vi "Autonomous Independent.vi"   [LabVIEW 2015]
doc: "This VI is called when autonomous begins, and will automatically be terminated when autonomous ends. You can carry out timed or sensor driven robot movement independently without needing to return to the caller."
uses:
  <vilib>/Rock Robotics/WPI/CAN/TalonSRX/WPI_CANTalonSRX_BrakeOverride.ctl
  <vilib>/Rock Robotics/WPI/Solenoid/WPI_SolenoidValue.ctl
  <vilib>/Analysis/baseanly.llb/Mean (DBL).vi
  <vilib>/Rock Robotics/WPI/Utilities/WPI_GetSetVariantRefNum.vi
  <vilib>/Rock Robotics/Network Tables/NT Write Numeric Array.vi
  <vilib>/Rock Robotics/Network Tables/NT Read Numeric Array.vi
  <vilib>/Rock Robotics/Network Tables/NT Read String Array.vi
  <vilib>/Rock Robotics/Network Tables/NT Write String.vi
  <vilib>/addons/control/pid/pid.llb/PID (DBL).vi
  <vilib>/Rock Robotics/WPI/Solenoid/WPI_SolenoidSetEnum.vi
  <vilib>/addons/control/pid/NI_PID_pid.lvlib
  ADI MXP IMU/ADI MXP IMU/FRC ADI MXP IMU.lvlib
  <vilib>/Analysis/NI_AALBase.lvlib
panel:
  # "Be sure to right-click and choose Data Operations>>Make Current Value default if you want to save the array values with the VI"
types:
  T1 = typedef "WPI_JoystickDevRef.ctl" = cluster{"Device":T2}
  T2 = typedef "WPI_JoystickDeviceEnum.ctl" = enum16{"USB 0", "USB 1", "USB 2", "USB 3", "USB 4", "USB 5"}
  T3 = typedef "WPI_EncoderDevRef.ctl" = cluster{"DevStatus":errorcluster, "EncoderIndex":T4, "CounterIndex":T5, "DistancePerCount":dbl, "Decoding Type":T6}
  T4 = typedef "FPGA_EncoderIdx.ctl" = enum8{"Enc 0", "Enc 1", "Enc 2", "Enc 3", "Enc 4", "Enc 5", "Enc 6", "Enc 7", "Invalid"}
  T5 = typedef "FPGA_CounterCtrSystemIndex.ctl" = enum8{"Ctr 0", "Ctr 1", "Ctr 2", "Ctr 3", "Ctr 4", "Ctr 5", "Ctr 6", "Ctr 7", "Invalid"}
  T6 = typedef "WPI_EncoderType.ctl" = enum16{"1x", "2x", "4x"}
  T7 = cluster{"proportional gain (Kc)":dbl, "integral time (Ti, min)":dbl, "derivative time (Td, min)":dbl}
  T8 = typedef "WPI_SolenoidValue.ctl" = enum16{"Off", "On", "Forward", "Reverse"}
  T9 = typedef "WPI_CANTalonSRX_BrakeOverride.ctl" = enum8{"No Override", "Override to Coast", "Override to Brake"}
  T10 = typedef "FRC ADI MXP IMU.lvlib/WPI_AnalogDevicesIMUInterruptDevRef.ctl" = cluster{"SimpleGyroDevRef":T11, "InterruptRef":T13}
  T11 = typedef "FRC ADI MXP IMU.lvlib/WPI_AnalogDevicesIMUDevRef.ctl" = cluster{"DevStatus":errorcluster, "Handle":i32, "SPI Bus":T12, "Device Found":bool, "Sample Rate":dbl, "Device Ready":bool, "Yaw Axis":enum16{"X", "Y", "Z"}, "AHRS Algorithm":enum16{"Complementary", "Madgwick"}}
  T12 = typedef "spi_bus.ctl" = enum16{"SPI On-Board, CS0", "SPI On-Board, CS1", "SPI On-Board, CS2", "SPI On-Board, CS3", "SPI MXP", "Invalid"}
  T13 = typedef "WPI_InterruptRef.ctl" = cluster{"DevStatus":errorcluster, "InterruptIndex":T14}
  T14 = typedef "FPGA_InterruptIndex.ctl" = enum8{"0", "1", "2", "3", "4", "5", "6", "7", "Invalid"}
  T15 = typedef "WPI_SolenoidDevRef.ctl" = cluster{"DevStatus":errorcluster, "Pneumatics Control Module":u8, "Forward Solenoid Channel":T16, "Reverse Solenoid Channel":T16}
  T16 = typedef "WPI_SolenoidChannel.ctl" = enum8{"Solenoid 0", "Solenoid 1", "Solenoid 2", "Solenoid 3", "Solenoid 4", "Solenoid 5", "Solenoid 6", "Solenoid 7", "Invalid"}
  T17 = typedef "WPI_MotorControlDeviceRef.ctl" = cluster{"DeviceStatus":errorcluster, "Type":T18, "PWM":cluster{"PWM Channel":T19, "DeadBand":T20}, "CAN":cluster{"Device Number":u8, "Control Mode":T21, "Semaphore":T22, "Max Vout":dbl, "TalonSRX Control Mode":T23}, "Invert":bool}
  T18 = typedef "WPI_MotorControlType.ctl" = enum16{"PWM", "CAN", "CANTalonSRX"}
  T19 = typedef "FPGA_DIOPWMChannel.ctl" = enum8{"PWM 0", "PWM 1", "PWM 2", "PWM 3", "PWM 4", "PWM 5", "PWM 6", "PWM 7", "PWM 8", "PWM 9", "PWM MXP 0", "PWM MXP 1", "PWM MXP 2", "PWM MXP 3", "PWM MXP 4", "PWM MXP 5", "PWM MXP 6", "PWM MXP 7", "PWM MXP 8", "PWM MXP 9", "Invalid"}
  T20 = typedef "WPI_PWMDeadband.ctl" = cluster{"Name":string, "maxPositivePwm":i32, "minPositivePwm":i32, "centerPwm":i32, "maxNegativePwm":i32, "minNegativePwm":i32, "angularRange":u16}
  T21 = typedef "WPI_CANJaguar_ControlMode.ctl" = enum8{"Percent VBus", "Current", "Speed", "Position", "Voltage"}
  T22 = typedef "Semaphore RefNum" = refnum<k1>
  T23 = typedef "WPI_CANTalonSRX_APIControlMode.ctl" = enum8{"Percent VBus", "Speed", "Position", "Slave", "Unchanged / Invalid", "Voltage Compensation", "Current", "Motion Profile"}
  T24 = cluster{"X Angle":dbl, "Y Angle":dbl, "Z Angle":dbl}
  T25 = typedef "WPI_SwitchDevRef.ctl" = cluster{"DevStatus":errorcluster, "DIO Channel":T26, "CntIndex":T5, "Normally Closed":bool}
  T26 = typedef "FPGA_DIOChannel.ctl" = enum8{"DIO 0", "DIO 1", "DIO 2", "DIO 3", "DIO 4", "DIO 5", "DIO 6", "DIO 7", "DIO 8", "DIO 9", "DIO MXP 0", "DIO MXP 1", "DIO MXP 2", "DIO MXP 3", "DIO MXP 4", "DIO MXP 5", "DIO MXP 6", "DIO MXP 7", "DIO MXP 8", "DIO MXP 9", "DIO MXP 10", "DIO MXP 11", "DIO MXP 12", "DIO MXP 13", "DIO MXP 14", "DIO MXP 15", "Invalid"}
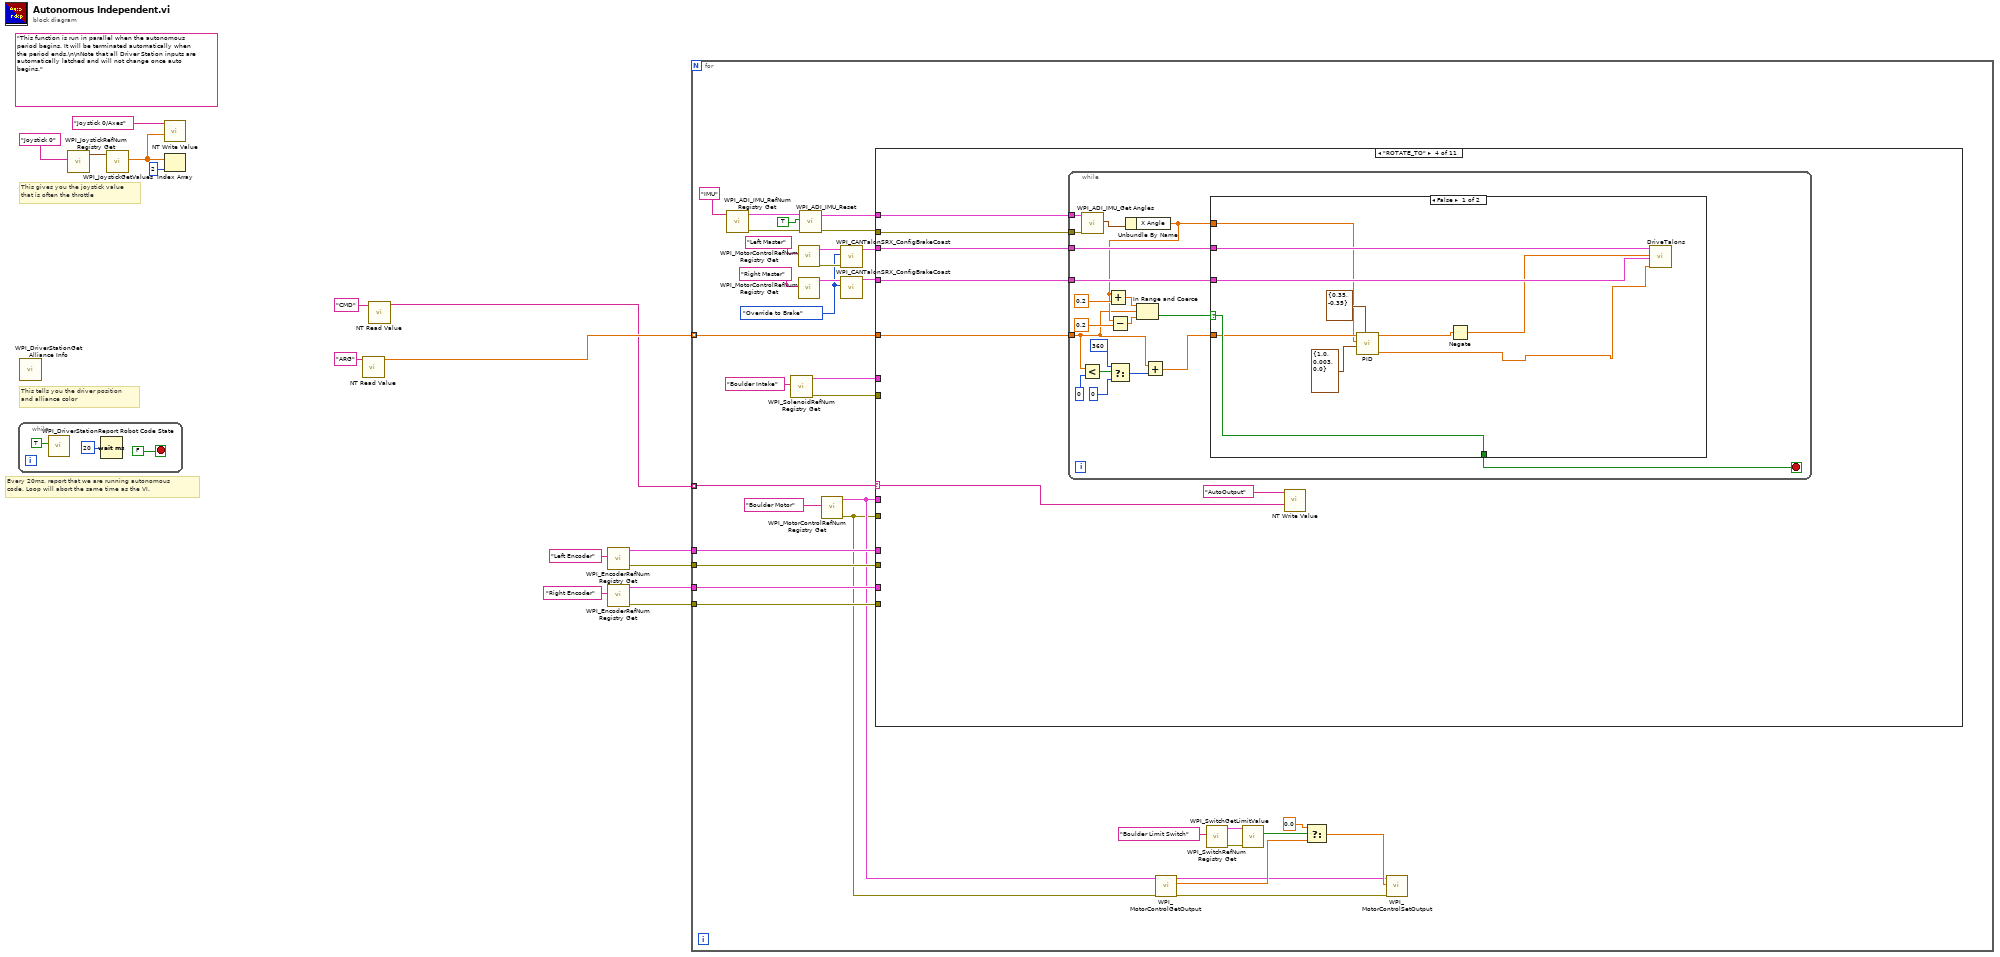
[diagram p0: block diagram]
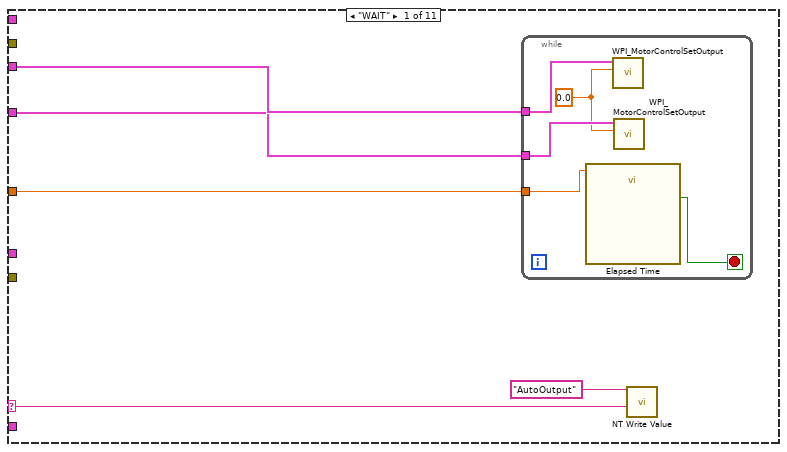
[diagram p2: hidden frame]
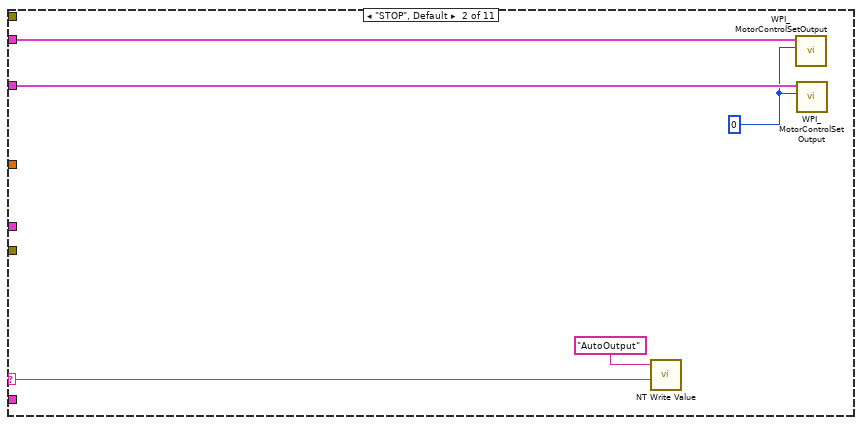
[diagram p3: hidden frame]
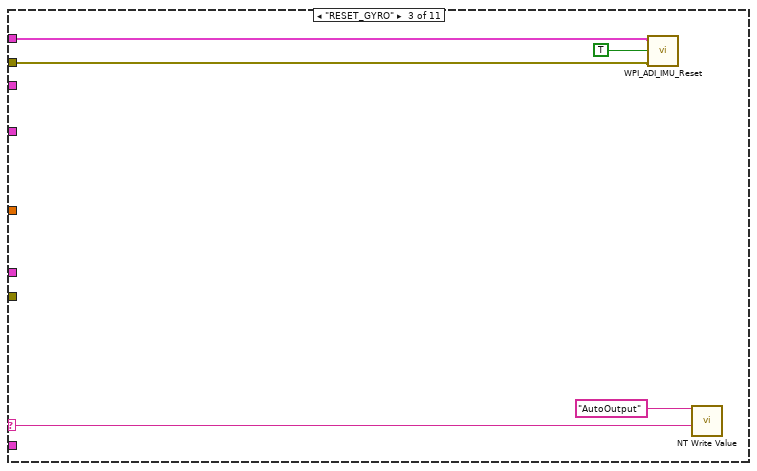
[diagram p4: hidden frame]
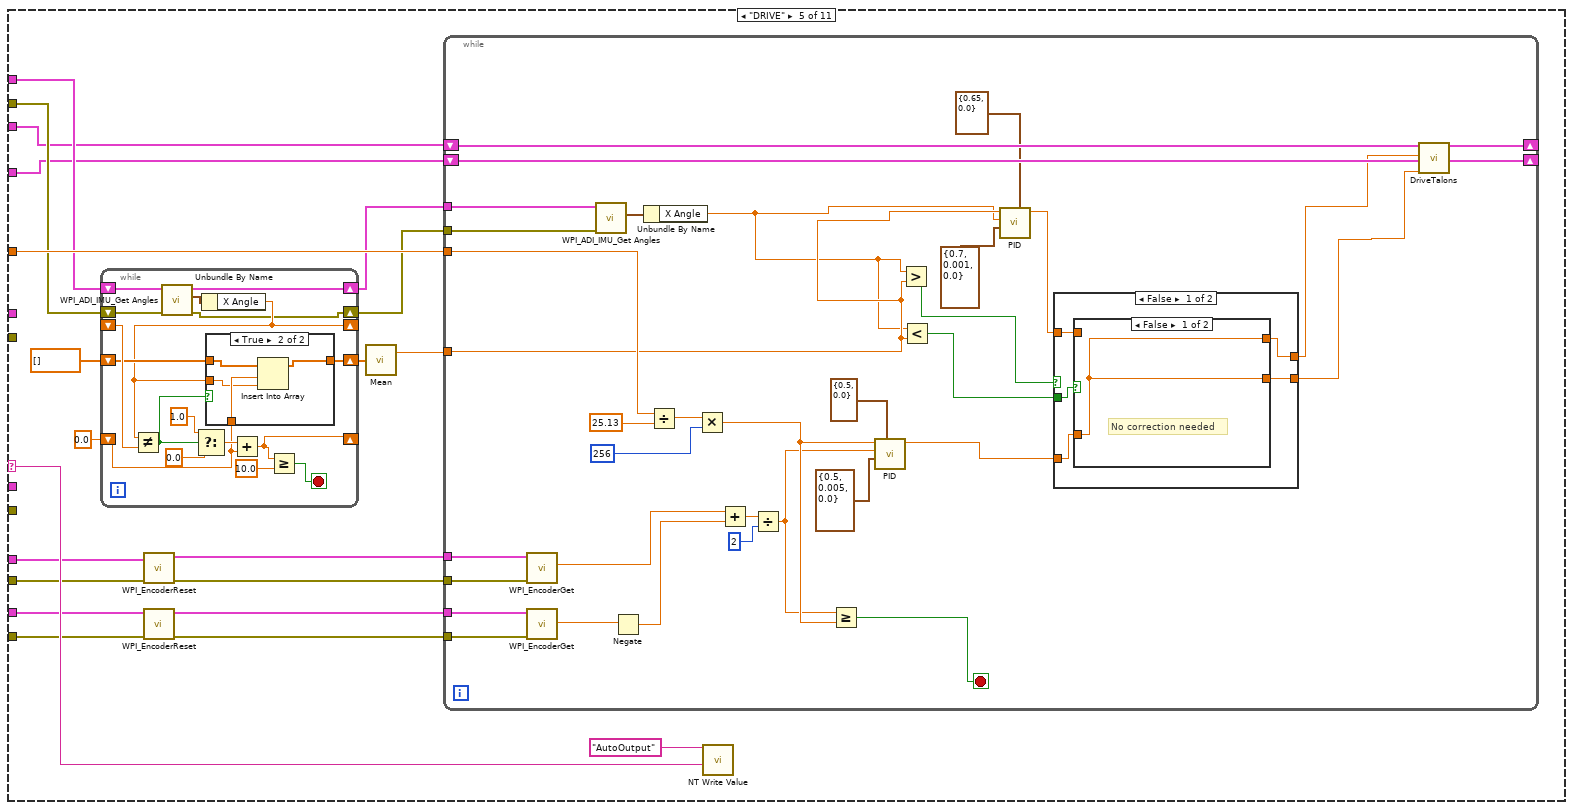
[diagram p6: hidden frame]
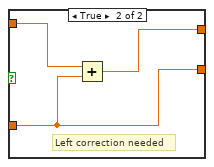
[diagram p8: hidden frame]
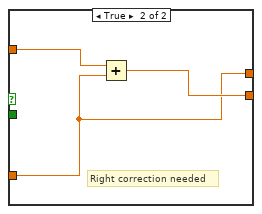
[diagram p9: hidden frame]
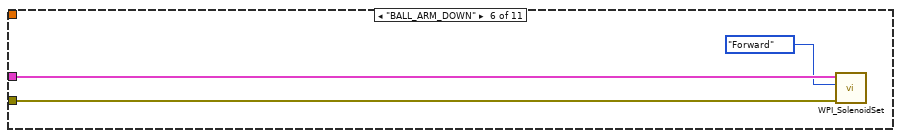
[diagram p10: hidden frame]
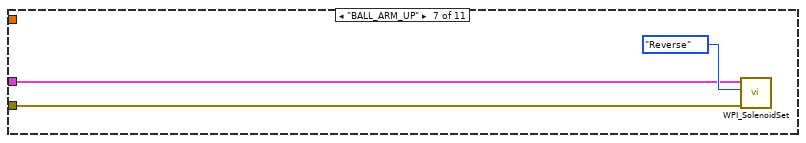
[diagram p11: hidden frame]
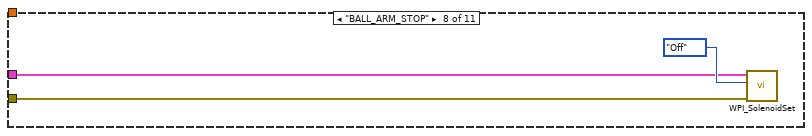
[diagram p12: hidden frame]
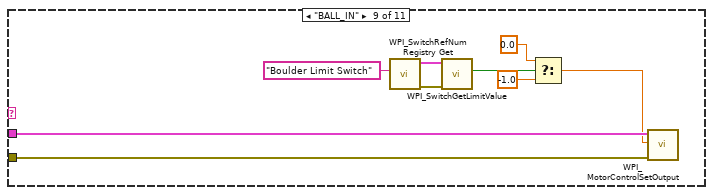
[diagram p13: hidden frame]
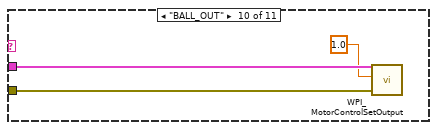
[diagram p14: hidden frame]
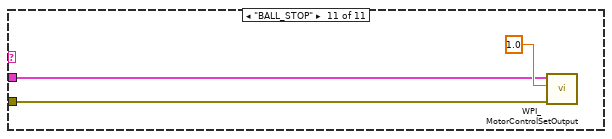
[diagram p15: hidden frame]
diagram:
  (unwired) "This function is run in parallel when the autonomous period begins. It will be terminated automatically when the period ends.\n\nNote that all Driver Station inputs are automatically latched and will not change once auto begins."
  # "Every 20ms, report that we are running autonomous\ncode. Loop will abort the same time as the VI."
  # "This gives you the joystick value\nthat is often the throttle"
  # "This tells you the driver position\nand alliance color"
  n1 = while {
    stop <- FALSE stop-if-true
    n2 = call <vilib>:"WPI_DriverStationReport Robot Code State.vi"("Autonomous"=TRUE) -> ()  [unwired: 10 in, 1 out]
    n3 = Wait (ms)(milliseconds to wait=u32 20) -> ()  [unwired: 1 out]
  }
  n4 = call <vilib>:"WPI_DriverStationGet Alliance Info.vi"() -> ()  [unwired: 12 out]
  n5 = call <vilib>:"WPI_JoystickRefNum Registry Get.vi"("refnum name"="Joystick 0") -> ("JoystickDevRef"=w14:T1)  [unwired: 1 in, 9 out]
  n6 = call <vilib>:"WPI_JoystickGetValues.vi"("JoystickDevRef"=w14) -> ("Axes"=w12:dbl[])  [unwired: 6 in, 4 out]
  n7 = call-poly <vilib>:"NT Write Value.vi"("Numeric Array"=w12, "Name"="Joystick 0/Axes") -> ()  [unwired: 9 in, 1 out]
  n8 = Index Array(array=w12, index=2) -> ()  [unwired: 1 out]
  n9 = call-poly <vilib>:"NT Read Value.vi"("Name"="ARG") -> ("Numeric Array"=w8:dbl[])  [unwired: 9 in, 1 out]
  n10 = call-poly <vilib>:"NT Read Value.vi"("Name"="CMD") -> ("String Array"=w7:string[])  [unwired: 9 in, 1 out]
  n11 = call <vilib>:"WPI_EncoderRefNum Registry Get.vi"("refnum name"="Left Encoder") -> ("error out"=w3:errorcluster, "EncoderDevRef"=w4:T3)  [unwired: 9 in]
  n12 = call <vilib>:"WPI_EncoderRefNum Registry Get.vi"("refnum name"="Right Encoder") -> ("error out"=w1:errorcluster, "EncoderDevRef"=w2:T3)  [unwired: 9 in]
  n13 = for {
    tunnel: w7 -> [w53] mode=indexing
    tunnel: w8 -> [w52] mode=indexing
    tunnel: w4 -> [w48]
    tunnel: w3 -> [w47]
    tunnel: w2 -> [w46]
    tunnel: w1 -> [w45]
    w39 = WPI_CANTalonSRX_BrakeOverride."Override to Brake" ("Brake / Coast Mode")
    n14 = call "WPI_ADI_IMU_RefNum Registry Get.vi"("refnum name"="IMU") -> ("error out"=w37:errorcluster, "ADI IMU Interrupt DevRef"=w38:T10)  [unwired: 9 in]
    n15 = call <vilib>:"WPI_SolenoidRefNum Registry Get.vi"("refnum name"="Boulder Intake") -> ("error out"=w31:errorcluster, "SolenoidDevRef"=w32:T15)  [unwired: 9 in]
    n16 = call <vilib>:"WPI_MotorControlRefNum Registry Get.vi"("refnum name"="Left Master") -> ("error out"=w42:errorcluster, "MotorControlDevRef"=w43:T17)  [unwired: 9 in]
    n17 = call <vilib>:"WPI_MotorControlRefNum Registry Get.vi"("refnum name"="Right Master") -> ("MotorControlDevRef"=w41:T17)  [unwired: 9 in, 1 out]
    n18 = call "WPI_ADI_IMU_Reset.vi"("error in"=w37, "Reset? (T)"=TRUE, "ADI IMU Interrupt DevRef"=w38) -> ("error out"=w36:errorcluster, "ADI IMU Interrupt DevRef Out"=w35:T10)  [unwired: 7 in]
    n19 = call <vilib>:"WPI_MotorControlRefNum Registry Get.vi"("refnum name"="Boulder Motor") -> ("error out"=w19:errorcluster, "MotorControlDevRef"=w20:T17)  [unwired: 9 in]
    n20 = call <vilib>:"WPI_CANTalonSRX_ConfigBrakeCoast.vi"("error in (no error)"=w42, "Brake / Coast Mode"=w39, "CAN Talon SRX Ref"=w43) -> ("CAN Talon SRX Ref"=w44:T17)  [unwired: 7 in, 1 out]
    n21 = call <vilib>:"WPI_CANTalonSRX_ConfigBrakeCoast.vi"("Brake / Coast Mode"=w39, "CAN Talon SRX Ref"=w41) -> ("CAN Talon SRX Ref"=w40:T17)  [unwired: 8 in, 1 out]
    n22 = case shown="\"ROTATE_TO\"" w53 {
      selector: w53 -> [w57 w67 w72 w76 w129 _ _ _ _ _ _]
      tunnel: w44 -> [w55 w66 _ w74 w114 _ _ _ _ _ _]
      tunnel: w52 -> [w56 _ _ w78 w130 _ _ _ _ _ _]
      tunnel: w35 -> [_ _ w71 w80 w120 _ _ _ _ _ _]
      tunnel: w36 -> [_ _ w70 w79 w118 _ _ _ _ _ _]
      tunnel: w40 -> [w54 w65 _ w75 w113 _ _ _ _ _ _]
      tunnel: w48 -> [_ _ _ _ w128 _ _ _ _ _ _]
      tunnel: w47 -> [_ _ _ _ w125 _ _ _ _ _ _]
      tunnel: w46 -> [_ _ _ _ w124 _ _ _ _ _ _]
      tunnel: w45 -> [_ _ _ _ w123 _ _ _ _ _ _]
      tunnel: w32 -> [_ _ _ _ _ w203 w205 w208 _ _ _]
      tunnel: w31 -> [_ _ _ _ _ w202 w204 w207 _ _ _]
      tunnel: w20 -> [_ _ _ _ _ _ _ _ w212 w221 w223]
      tunnel: w19 -> [_ _ _ _ _ _ _ _ w211 w220 w222]
      frame "WAIT" {
        n23 = while {
          tunnel: w56 -> [w63]
          tunnel: w55 -> [w61]
          tunnel: w54 -> [w60]
          stop <- w62 stop-if-true
          w59 = 0.0
          n24 = call "Elapsed Time"("Time Target (s)"=w63) -> ("Time has Elapsed"=w62:bool)  [unwired: 11 in, 7 out]
          n25 = call <vilib>:"WPI_MotorControlSetOutput.vi"("Output"=w59, "MotorControlDevRef"=w61) -> ()  [unwired: 7 in, 3 out]
          n26 = call <vilib>:"WPI_MotorControlSetOutput.vi"("Output"=w59, "MotorControlDevRef"=w60) -> ()  [unwired: 7 in, 3 out]
        }
        n27 = call-poly <vilib>:"NT Write Value.vi"("String"=w57, "Name"="AutoOutput") -> ()  [unwired: 9 in, 1 out]
      }
      frame "STOP", Default {
        w64 = 0
        n28 = call-poly <vilib>:"NT Write Value.vi"("String"=w67, "Name"="AutoOutput") -> ()  [unwired: 9 in, 1 out]
        n29 = call <vilib>:"WPI_MotorControlSetOutput.vi"("Output"=w64, "MotorControlDevRef"=w66) -> ()  [unwired: 7 in, 3 out]
        n30 = call <vilib>:"WPI_MotorControlSetOutput.vi"("Output"=w64, "MotorControlDevRef"=w65) -> ()  [unwired: 7 in, 3 out]
      }
      frame "RESET_GYRO" {
        n31 = call "WPI_ADI_IMU_Reset.vi"("error in"=w70, "Reset? (T)"=TRUE, "ADI IMU Interrupt DevRef"=w71) -> ()  [unwired: 7 in, 2 out]
        n32 = call-poly <vilib>:"NT Write Value.vi"("String"=w72, "Name"="AutoOutput") -> ()  [unwired: 9 in, 1 out]
      }
      frame "ROTATE_TO" {
        n33 = while {
          tunnel: w80 -> [w83]
          tunnel: w79 -> [w82]
          tunnel: w78 -> [w85]
          tunnel: w75 -> [w90]
          tunnel: w74 -> [w89]
          stop <- w99 stop-if-true
          n34 = Less?(x=w85, y=0) -> (x < y?=w94:bool)
          n35 = call "WPI_ADI_IMU_Get Angles.vi"("error in"=w82, "ADI IMU Interrupt DevRef"=w83) -> ("IMU Angles"=w81:T24)  [unwired: 6 in, 3 out]
          n36 = Select(t=360, s=w94, f=0) -> (s? t:f=w87:i32)
          n37 = Unbundle By Name(w81) -> ("X Angle"=w88:dbl)
          n38 = Add(x=w88, y=0.2) -> (x+y=w97:dbl)
          n39 = Subtract(x=w88, y=0.2) -> (x-y=w95:dbl)
          n40 = In Range and Coerce(upper limit=w97, x=w85, lower limit=w95) -> (In Range?=w84:bool)  [unwired: 1 out]
          n41 = Add(x=w85, y=w87) -> (x+y=w86:dbl)
          n42 = case shown="False" w84 {
            selector: w84 -> [w107 w110]
            tunnel: w86 -> [w106 _]
            tunnel: [w107 w110] -> w99
            tunnel: w88 -> [w103 _]
            tunnel: w90 -> [w104 _]
            tunnel: w89 -> [w105 _]
            frame False {
              n43 = call-poly <vilib>:"PID.vi"("output range"=cluster{"output high":dbl, "output low":dbl} {"output high"=0.35, "output low"=-0.35}, "PID gains"=T7 {"proportional gain (Kc)"=1.0, "integral time (Ti, min)"=0.003, "derivative time (Td, min)"=0.0}, "process variable"=w103, "setpoint"=w106) -> ("dt out (s)"=w100:dbl, "output"=w102:dbl)  [unwired: 6 in]
              n44 = Negate(x=w102) -> (-x=w101:dbl)
              n45 = call "DriveTalons.vi"("Left Motor"=w105, "Left Stick"=w101, "Right Motor"=w104, "Right Stick"=w100) -> ()  [unwired: 12 in, 4 out]
            }
            frame True {
            }
          }
        }
        n46 = call-poly <vilib>:"NT Write Value.vi"("String"=w76, "Name"="AutoOutput") -> ()  [unwired: 9 in, 1 out]
      }
      frame "DRIVE" {
        n47 = while {
          shift-right: [w139] -> _
          shift-left: _ -> [w148]
          shift-right: [w140] -> _
          shift-left: 0.0 -> [w137]
          shift-right: [w134] -> w119
          shift-left: w120 -> [w135]
          shift-right: [w132] -> w117
          shift-left: w118 -> [w136]
          shift-right: [w138] -> w115
          shift-left: dbl[] [] -> [w141]
          stop <- w144 stop-if-true
          n48 = call "WPI_ADI_IMU_Get Angles.vi"("error in"=w136, "ADI IMU Interrupt DevRef"=w135) -> ("error out"=w132:errorcluster, "IMU Angles"=w133:T24, "ADI IMU Interrupt DevRef Out"=w134:T10)  [unwired: 6 in, 1 out]
          n49 = Unbundle By Name(w133) -> ("X Angle"=w139:dbl)
          n50 = Not Equal?(x=w139, y=w148) -> (x != y?=w142:bool)
          n51 = Select(t=1.0, s=w142, f=0.0) -> (s? t:f=w145:dbl)
          n52 = case shown="True" w142 {
            tunnel: w141 -> [w149 w153]
            tunnel: [w149 w152] -> w138
            tunnel: w139 -> [_ w150]
            tunnel: w137 -> [_ w151]
            frame False {
            }
            frame True {
              n53 = Insert Into Array(array=w153, index=w151, new element=w150) -> (w152:dbl[])
            }
          }
          n54 = Add(x=w145, y=w137) -> (x+y=w140:dbl)
          n55 = Greater Or Equal?(x=w140, y=10.0) -> (x >= y?=w144:bool)
        }
        n56 = call <vilib>:"WPI_EncoderReset.vi"("error in (no error)"=w125, "EncoderDevRef"=w128) -> ("error out"=w126:errorcluster, "EncoderDevRef"=w127:T3)  [unwired: 8 in]
        n57 = call <vilib>:"WPI_EncoderReset.vi"("error in (no error)"=w123, "EncoderDevRef"=w124) -> ("error out"=w121:errorcluster, "EncoderDevRef"=w122:T3)  [unwired: 8 in]
        n58 = call-poly <vilib>:"Mean.vi"("X"=w115) -> ("mean"=w111:dbl)  [unwired: 1 out]
        n59 = while {
          tunnel: w130 -> [w186]
          tunnel: w127 -> [w180]
          tunnel: w126 -> [w179]
          tunnel: w122 -> [w178]
          tunnel: w121 -> [w177]
          tunnel: w119 -> [w159]
          tunnel: w117 -> [w158]
          shift-right: [w170] -> _
          shift-left: w114 -> [w182]
          shift-right: [w169] -> _
          shift-left: w113 -> [w181]
          tunnel: w111 -> [w161]
          stop <- w176 stop-if-true
          n60 = call <vilib>:"WPI_EncoderGet.vi"("error in (no error)"=w179, "EncoderDevRef"=w180) -> ("Distance"=w168:dbl)  [unwired: 4 in, 5 out]
          n61 = call <vilib>:"WPI_EncoderGet.vi"("error in (no error)"=w177, "EncoderDevRef"=w178) -> ("Distance"=w166:dbl)  [unwired: 4 in, 5 out]
          n62 = call "WPI_ADI_IMU_Get Angles.vi"("error in"=w158, "ADI IMU Interrupt DevRef"=w159) -> ("IMU Angles"=w157:T24)  [unwired: 6 in, 3 out]
          n63 = Negate(x=w166) -> (-x=w167:dbl)
          n64 = Unbundle By Name(w157) -> ("X Angle"=w156:dbl)
          n65 = Divide(x=w186, y=25.13) -> (x/y=w184:dbl)
          n66 = Multiply(x=w184, y=256) -> (x*y=w175:dbl)
          n67 = Add(x=w168, y=w167) -> (x+y=w188:dbl)
          n68 = Divide(x=w188, y=2) -> (x/y=w174:dbl)
          n69 = Greater Or Equal?(x=w174, y=w175) -> (x >= y?=w176:bool)
          n70 = call-poly <vilib>:"PID.vi"("output range"=cluster{"output high":dbl, "output low":dbl} {"output high"=0.5, "output low"=0.0}, "PID gains"=T7 {"proportional gain (Kc)"=0.5, "integral time (Ti, min)"=0.005, "derivative time (Td, min)"=0.0}, "process variable"=w174, "setpoint"=w175) -> ("output"=w173:dbl)  [unwired: 6 in, 1 out]
          n71 = Greater?(x=w156, y=w161) -> (0:w172:bool)
          n72 = Less?(x=w156, y=w161) -> (x < y?=w171:bool)
          n73 = call-poly <vilib>:"PID.vi"("output range"=cluster{"output high":dbl, "output low":dbl} {"output high"=0.65, "output low"=0.0}, "PID gains"=T7 {"proportional gain (Kc)"=0.7, "integral time (Ti, min)"=0.001, "derivative time (Td, min)"=0.0}, "process variable"=w156, "setpoint"=w161) -> ("output"=w160:dbl)  [unwired: 6 in, 1 out]
          n74 = case shown="False" w172 {
            tunnel: w160 -> [w193 w199]
            tunnel: [w189 w198] -> w155
            tunnel: [w191 w200] -> w154
            tunnel: w173 -> [w190 w198]
            tunnel: w171 -> [w192 _]
            frame False {
              n75 = case shown="False" w192 {
                tunnel: [w194 w197] -> w189
                tunnel: w193 -> [_ w196]
                tunnel: [w194 w195] -> w191
                tunnel: w190 -> [w194 w195]
                frame False {
                  # "No correction needed"
                }
                frame True {
                  # "Left correction needed"
                  n76 = Add(x=w196, y=w195) -> (x+y=w197:dbl)
                }
              }
            }
            frame True {
              # "Right correction needed"
              n77 = Add(x=w199, y=w198) -> (x+y=w200:dbl)
            }
          }
          n78 = call "DriveTalons.vi"("Left Motor"=w182, "Left Stick"=w155, "Right Motor"=w181, "Right Stick"=w154) -> ("Left Motor Out"=w170:T17, "Right Motor Out"=w169:T17)  [unwired: 12 in, 2 out]
        }
        n79 = call-poly <vilib>:"NT Write Value.vi"("String"=w129, "Name"="AutoOutput") -> ()  [unwired: 9 in, 1 out]
      }
      frame "BALL_ARM_DOWN" {
        n80 = call-poly <vilib>:"WPI_SolenoidSet.vi"("error in (no error)"=w202, "Value"=WPI_SolenoidValue."Forward", "SolenoidDevRef"=w203) -> ()  [unwired: 7 in, 2 out]
      }
      frame "BALL_ARM_UP" {
        n81 = call-poly <vilib>:"WPI_SolenoidSet.vi"("error in (no error)"=w204, "Value"=WPI_SolenoidValue."Reverse", "SolenoidDevRef"=w205) -> ()  [unwired: 7 in, 2 out]
      }
      frame "BALL_ARM_STOP" {
        n82 = call-poly <vilib>:"WPI_SolenoidSet.vi"("error in (no error)"=w207, "Value"=WPI_SolenoidValue."Off", "SolenoidDevRef"=w208) -> ()  [unwired: 7 in, 2 out]
      }
      frame "BALL_IN" {
        n83 = call <vilib>:"WPI_SwitchRefNum Registry Get.vi"("refnum name"="Boulder Limit Switch") -> ("error out"=w217:errorcluster, "SwitchDevRef"=w216:T25)  [unwired: 9 in]
        n84 = call <vilib>:"WPI_SwitchGetLimitValue.vi"("error in (no error)"=w217, "SwitchDevRef"=w216) -> ("Switch Pressed"=w215:bool)  [unwired: 7 in, 2 out]
        n85 = Select(t=0.0, s=w215, f=-1.0) -> (s? t:f=w210:dbl)
        n86 = call <vilib>:"WPI_MotorControlSetOutput.vi"("error in (no error)"=w211, "Output"=w210, "MotorControlDevRef"=w212) -> ()  [unwired: 6 in, 3 out]
      }
      frame "BALL_OUT" {
        n87 = call <vilib>:"WPI_MotorControlSetOutput.vi"("error in (no error)"=w220, "Output"=1.0, "MotorControlDevRef"=w221) -> ()  [unwired: 6 in, 3 out]
      }
      frame "BALL_STOP" {
        n88 = call <vilib>:"WPI_MotorControlSetOutput.vi"("error in (no error)"=w222, "Output"=1.0, "MotorControlDevRef"=w223) -> ()  [unwired: 6 in, 3 out]
      }
    }
    n89 = call <vilib>:"WPI_MotorControlGetOutput.vi"("error in (no error)"=w19, "MotorControlDevRef"=w20) -> ("error out"=w21:errorcluster, "Output"=w23:dbl, "MotorControlDevRef"=w22:T17)  [unwired: 7 in]
    n90 = call <vilib>:"WPI_SwitchRefNum Registry Get.vi"("refnum name"="Boulder Limit Switch") -> ("error out"=w28:errorcluster, "SwitchDevRef"=w27:T25)  [unwired: 9 in]
    n91 = call <vilib>:"WPI_SwitchGetLimitValue.vi"("error in (no error)"=w28, "SwitchDevRef"=w27) -> ("Switch Pressed"=w26:bool)  [unwired: 7 in, 2 out]
    n92 = Select(t=0.0, s=w26, f=w23) -> (s? t:f=w24:dbl)
    n93 = call <vilib>:"WPI_MotorControlSetOutput.vi"("error in (no error)"=w21, "Output"=w24, "MotorControlDevRef"=w22) -> ()  [unwired: 6 in, 3 out]
  }
